vi "Set CD Name.vi"(10 "CD Name":string, 11 "Project XML Editor in":refnum<class "Project XML Editor.lvclass">) -> (3 "Project XML Editor out":refnum<class "Project XML Editor.lvclass">)   [LabVIEW 2018, in ".LVLIBP CD XML Updater.lvlib" / "Project XML Editor.lvclass"]
uses:
  Project XML Editor.lvclass
  Project XML Editor.lvclass/Project XML Editor.ctl
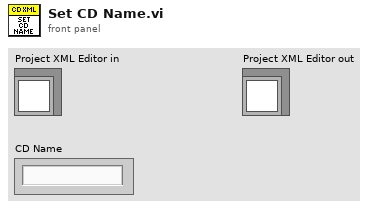
[diagram p1: front panel]
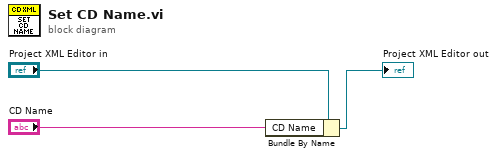
[diagram p0: block diagram]
diagram:
  n1 = Bundle By Name(cluster="Project XML Editor in", "CD Name"="CD Name") -> (→"Project XML Editor out":refnum<class "Project XML Editor.lvclass">)
